vi "checkForNewImages.vi"(8 "error in (no error)":errorcluster, 11 "ImagesToQueue in":refnum<class "ImagesToQueue.lvclass">) -> (0 "error out":errorcluster, 3 "ImagesToQueue out":refnum<class "ImagesToQueue.lvclass">)   [LabVIEW 2011, in "Views.lvlib" / "Camera.lvlib" / "ImagesToQueue.lvclass"]
uses:
  ImagesToQueue.lvclass
  Tools/Filing/FileNeologist/FileNeologist.lvclass
panel:
  in  "stop":bool
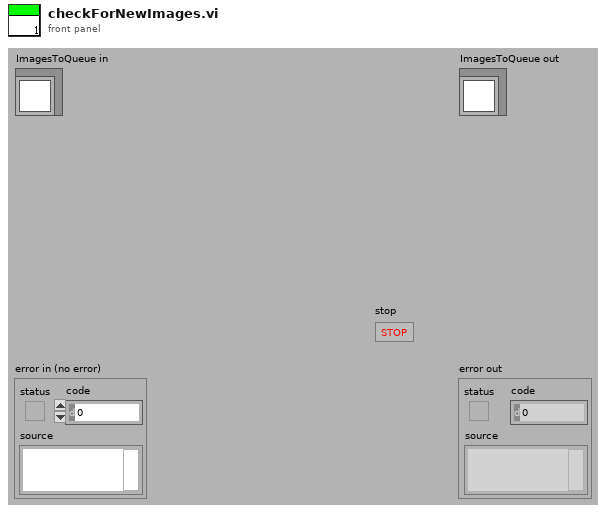
[diagram p1: front panel]
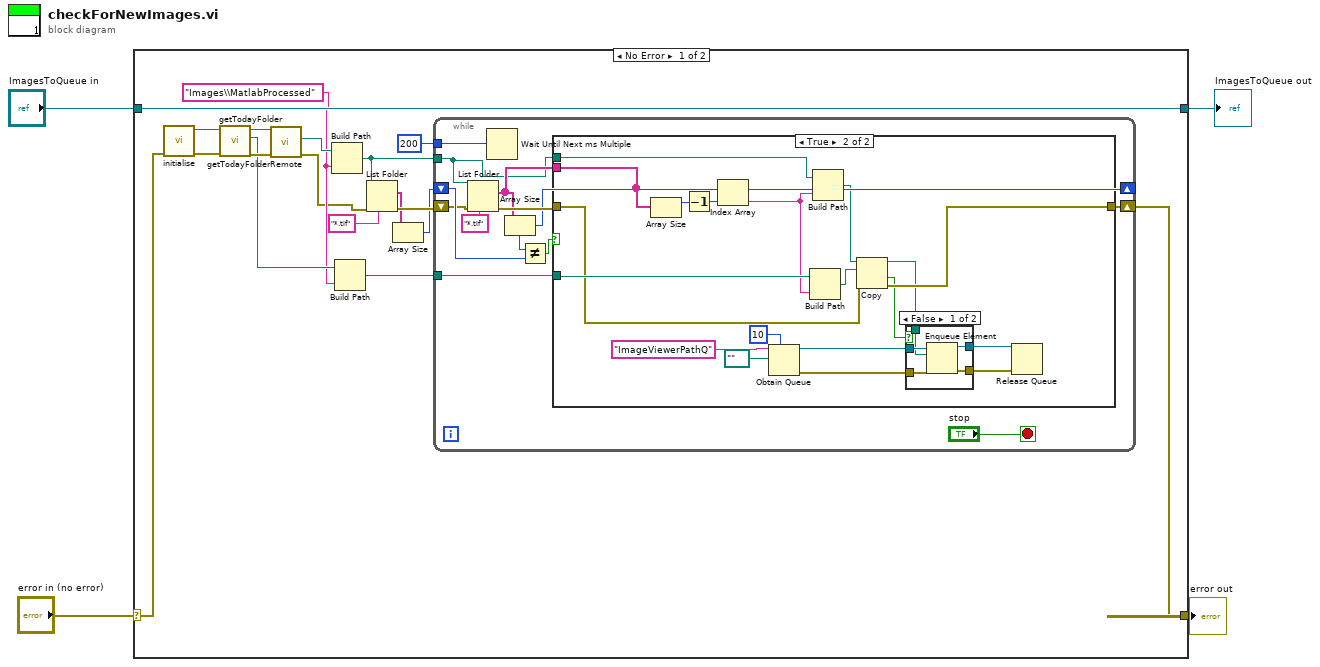
[diagram p0: block diagram]
diagram:
  n1 = case shown="No Error" "error in (no error)" {
    selector: "error in (no error)" -> [w21 w63]
    tunnel: [w12 w63] -> w3
    tunnel: [w22 w62] -> w1
    tunnel: "ImagesToQueue in" -> [w22 w62]
    frame No Error {
      w14 = "Images\\MatlabProcessed"
      n2 = call "initialise.vi"("error in (no error)"=w21) -> ("error out"=w16:errorcluster, "FileNeologist out"=w19:refnum<class "FileNeologist.lvclass">)  [unwired: 9 in]
      n3 = call "getTodayFolder.vi"("error in (no error)"=w16, "FileNeologist in"=w19) -> ("error out"=w17:errorcluster, "todayFolder"=w15:path, "FileNeologist out"=w18:refnum<class "FileNeologist.lvclass">)  [unwired: 7 in]
      n4 = call "getTodayFolderRemote.vi"("error in (no error)"=w17, "FileNeologist in"=w18) -> ("error out"=w7:errorcluster, "todayFolder"=w20:path)  [unwired: 7 in, 1 out]
      n5 = Build Path(base path=w20, name or relative path=w14) -> (appended path=w9:path)
      n6 = Build Path(base path=w15, name or relative path=w14) -> (appended path=w13:path)
      n7 = List Folder(path=w9, pattern="*.tif", error in=w7) -> (filenames=w5:string[], error out=w10:errorcluster)  [unwired: 1 in, 2 out]
      n8 = Array Size(array=w5) -> (size(s)=w6:i32)
      n9 = while {
        tunnel: w9 -> [w23]
        tunnel: w13 -> [w32]
        shift-right: [w31] -> w12
        shift-left: w10 -> [w26]
        shift-right: [w25] -> _
        shift-left: w6 -> [w34]
        tunnel: 200 -> [w29]
        stop <- "stop" stop-if-true
        n10 = List Folder(path=w23, pattern="*.tif", error in=w26) -> (filenames=w24:string[], error out=w28:errorcluster)  [unwired: 1 in, 2 out]
        n11 = Wait Until Next ms Multiple(millisecond multiple=w29) -> ()  [unwired: 1 out]
        n12 = Array Size(array=w24) -> (size(s)=w25:i32)
        n13 = Not Equal?(x=w25, y=w34) -> (x != y?=w33:bool)
        n14 = case shown="True" w33 {
          tunnel: w32 -> [_ w52]
          tunnel: w28 -> [w35 w39]
          tunnel: [w35 w50] -> w31
          tunnel: w24 -> [_ w40]
          tunnel: w23 -> [_ w38]
          frame False {
          }
          frame True {
            n15 = Array Size(array=w40) -> (size(s)=w54:i32)
            n16 = Decrement(x=w54) -> (x-1=w53:i32)
            n17 = Index Array(array=w40, index=w53) -> (element=w37:string)
            n18 = Obtain Queue(max queue size (-1, unlimited)=10, name (unnamed)="ImageViewerPathQ", element data type=path "") -> (queue out=w46:refnum<queue>, error out=w45:errorcluster)  [unwired: 2 in, 1 out]
            n19 = Build Path(base path=w52, name or relative path=w37) -> (appended path=w51:path)
            n20 = Build Path(base path=w38, name or relative path=w37) -> (appended path=w36:path)
            n21 = Copy(8:w39, 10:w51, 11:w36) -> (0:w50:errorcluster, 1:w43:bool, 3:w44:path)  [unwired: 2 in]
            n22 = case shown="False" w43 {
              tunnel: w46 -> [w59 w61]
              tunnel: w45 -> [w58 w60]
              tunnel: w44 -> [w57 _]
              tunnel: [w56 w61] -> w42
              tunnel: [w55 w60] -> w41
              frame False {
                n23 = Enqueue Element(queue=w59, element=w57, error in (no error)=w58) -> (queue out=w56:refnum<queue>, error out=w55:errorcluster)  [unwired: 1 in, 1 out]
              }
              frame True {
              }
            }
            n24 = Release Queue(queue=w42, error in (no error)=w41) -> ()  [unwired: 1 in, 3 out]
          }
        }
      }
    }
    frame Error {
    }
  }
  "error out" <- w3
  "ImagesToQueue out" <- w1
